vi "database operation using string.vi"() -> ()   [LabVIEW 2024]
panel:
  in  "Name":string
  in  "Password":string
  in  "Table Control":string[][](table)
  out "User Name":string
  out "Access Denied":bool
  out "Acess Given":bool
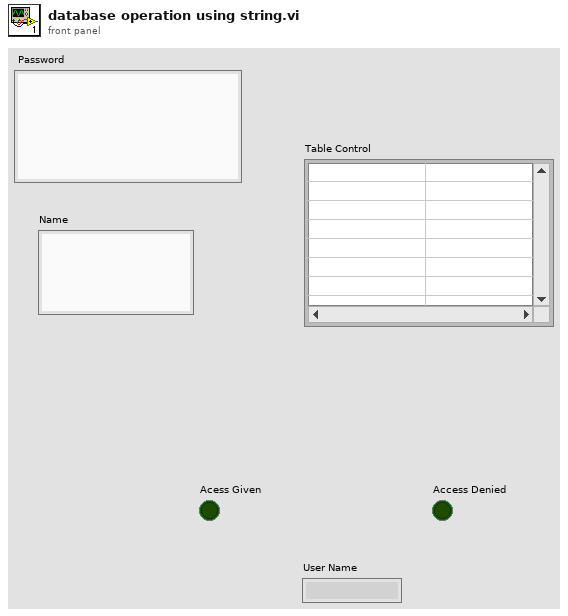
[diagram p1: front panel]
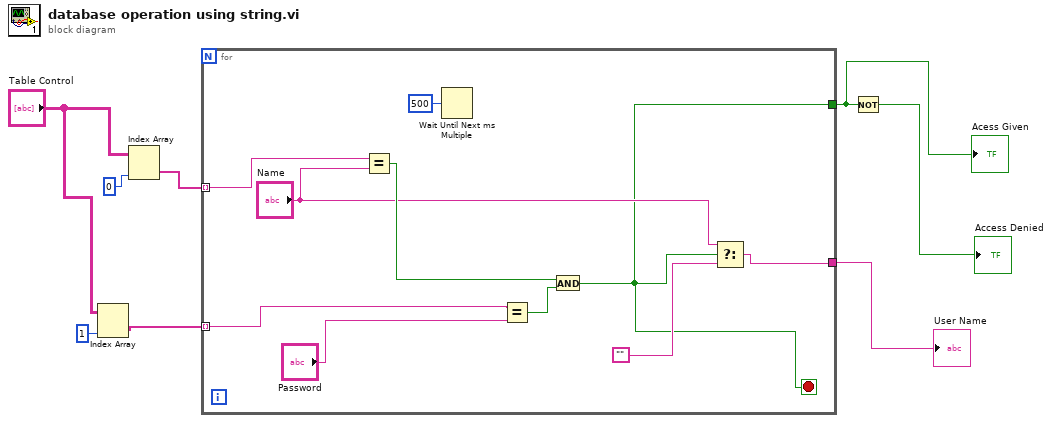
[diagram p0: block diagram]
diagram:
  n1 = Index Array(array="Table Control", index (col)=1 ("disabled index (col)")) -> (element=w6:string[])  [unwired: 1 in]
  n2 = Index Array(array="Table Control", index (col)=0 ("disabled index (col)")) -> (element=w7:string[])  [unwired: 1 in]
  n3 = for {
    tunnel: w7 -> [w13] mode=indexing
    tunnel: w6 -> [w10] mode=indexing
    tunnel: [w12] -> w5
    tunnel: [w9] -> w1
    stop <- w9 stop-if-true
    n4 = Equal?(x=w13, y="Name") -> (x = y?=w17:bool)
    n5 = Wait Until Next ms Multiple(millisecond multiple=u32 500) -> ()  [unwired: 1 out]
    n6 = Equal?(x=w10, y="Password") -> (x = y?=w16:bool)
    n7 = And(x=w17, y=w16) -> (x .and. y?=w9:bool)
    n8 = Select(t="Name", s=w9, f="") -> (s? t:f=w12:string)
  }
  "Acess Given" <- w1
  "User Name" <- w5
  n9 = Not(x=w1) -> (.not. x?=→"Access Denied":bool)
